vi "SetCheckedStatus.vi"(8 "error in (no error)":errorcluster, 9 "Checked":bool, 10 "MenuItem":refnum<class "MGI_MenuItem.lvclass">, 11 "MenuStrip in":refnum<class "MGI_MenuStrip.lvclass">) -> (0 "error out":errorcluster, 3 "MenuStrip out":refnum<class "MGI_MenuStrip.lvclass">)   [LabVIEW 2016, in "MGI_MenuStrip.lvclass"]
doc: "Sets the checked Status. Required to be overridden.\n\nAuthored by Derek E. Trepanier\nsupport@mooregoodideas.com\nwww.mooregoodideas.com\n\nCopyright (c) 2012, Moore Good Ideas, Inc.\n\nAll rights reserved.\n\nRedistribution and use in source and binary forms, with or without modification, are permitted provided that the following conditions are met:\n\n * Redistributions of source code must retain the above copyright notice, this list of conditions and the following disclaimer.\n * Redistributions in binary form must reproduce the above copyright notice, this list of conditions and the following disclaimer in the documentation and/or other materials provided with the distribution.\n * Neither the name of Moore Good Ideas, Inc. nor the names of its contributors may be used to endorse or promote products derived from this software without specific prior written permission.\n\nTHIS SOFTWARE IS PROVIDED BY THE COPYRIGHT HOLDERS AND CONTRIBUTORS \"AS IS\" AND ANY EXPRESS OR IMPLIED WARRANTIES, INCLUDING, BUT NOT LIMITED TO, THE IMPLIED WARRANTIES OF MERCHANTABILITY AND FITNESS FOR A PARTICULAR PURPOSE ARE DISCLAIMED. IN NO EVENT SHALL THE COPYRIGHT OWNER OR CONTRIBUTORS BE LIABLE FOR ANY DIRECT, INDIRECT, INCIDENTAL, SPECIAL, EXEMPLARY, OR CONSEQUENTIAL DAMAGES (INCLUDING, BUT NOT LIMITED TO, PROCUREMENT OF SUBSTITUTE GOODS OR SERVICES; LOSS OF USE, DATA, OR PROFITS; OR BUSINESS INTERRUPTION) HOWEVER CAUSED AND ON ANY THEORY OF LIABILITY, WHETHER IN CONTRACT, STRICT LIABILITY, OR TORT (INCLUDING NEGLIGENCE OR OTHERWISE) ARISING IN ANY WAY OUT OF THE USE OF THIS SOFTWARE, EVEN IF ADVISED OF THE POSSIBILITY OF SUCH DAMAGE."
uses:
  <userlib>/_MGI/Menu Building/MenuTypes/MenuStrip/MGI_MenuStrip.lvclass
  <userlib>/_MGI/Menu Building/MenuItem/MGI_MenuItem.lvclass
  System.Windows.Forms
  <userlib>/_MGI/Menu Building/MenuItem/Read Full Tag.vi
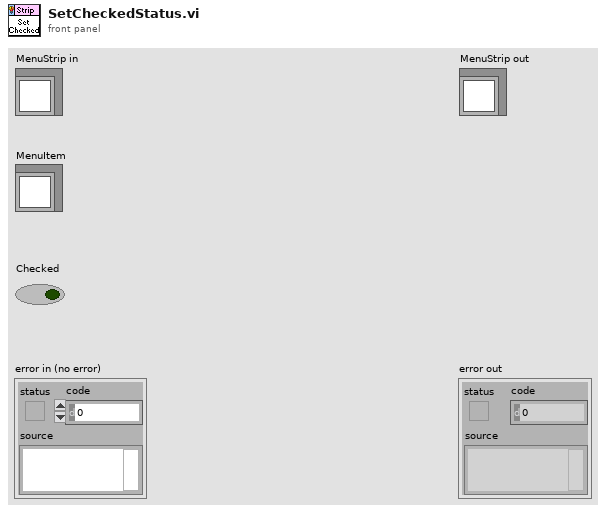
[diagram p1: front panel]
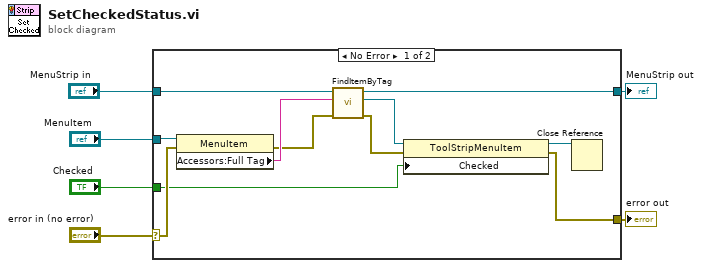
[diagram p0: block diagram]
diagram:
  n1 = case shown="No Error" "error in (no error)" {
    selector: "error in (no error)" -> [w12 w18]
    tunnel: [w9 w18] -> w2
    tunnel: [w14 w19] -> w5
    tunnel: "MenuStrip in" -> [w17 w19]
    tunnel: "MenuItem" -> [w16 _]
    tunnel: "Checked" -> [w8 _]
    frame No Error {
      n2 = property class="MenuItem"(reference=w16, error in=w12) -> (error out=w11:errorcluster, "Accessors:Full Tag"=w15:string)  [unwired: 1 out]
      n3 = call <userlib>:"FindItemByTag.vi"("error in (no error)"=w11, "Tag"=w15, "MenuStrip in"=w17) -> ("error out"=w10:errorcluster, "Tool Strip Menu Item"=w13:refnum<k24>, "MenuStrip out"=w14:refnum<class "MGI_MenuStrip.lvclass">)  [unwired: 6 in]
      n4 = property class="ToolStripMenuItem"(reference=w13, error in=w10, "Checked"=w8) -> (reference out=w7:refnum<k24>, error out=w9:errorcluster)
      n5 = Close Reference(reference=w7) -> ()  [unwired: 1 in, 1 out]
    }
    frame Error {
    }
  }
  "error out" <- w2
  "MenuStrip out" <- w5
